vi "Destroy.vi"(8 "error in (no error)":errorcluster, 11 "QueueMessenger in":refnum<class "QueueMessenger.lvclass">) -> (0 "error out":errorcluster)   [LabVIEW 2011, in "Messenging.lvlib" / "QueueMessenger.lvclass"]
uses:
  QueueMessenger.lvclass
  QueueMessenger.lvclass/QueueMessenger.ctl
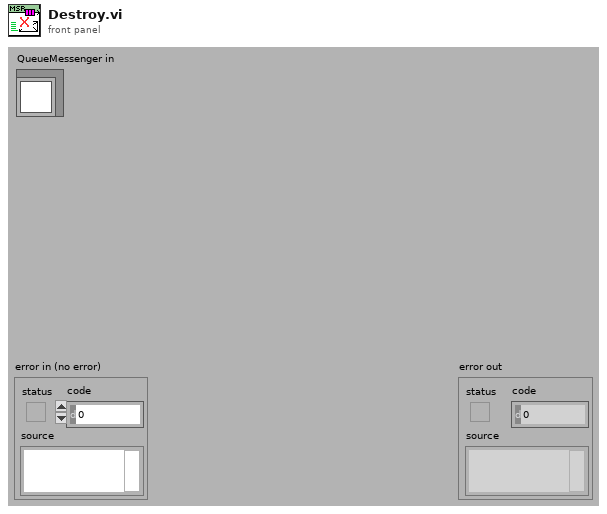
[diagram p1: front panel]
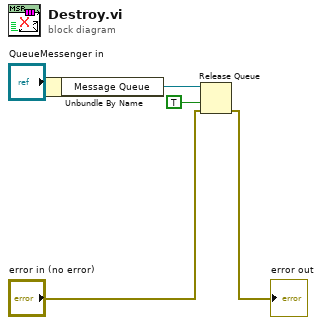
[diagram p0: block diagram]
diagram:
  n1 = Unbundle By Name("QueueMessenger in") -> ("Message Queue"=w4:refnum<queue>)
  n2 = Release Queue(queue=w4, force destroy? (F)=TRUE, error in (no error)="error in (no error)") -> (error out=→"error out":errorcluster)  [unwired: 2 out]
